vi "Create.vi"(8 "error in (no error)":errorcluster) -> (0 "error out":errorcluster, 3 "GH2 out":refnum<class "GH2.lvclass">)   [LabVIEW 2026, in "GH2.lvclass"]
uses:
  GH2.lvclass
  GH2.lvclass/GH2.ctl
  System.Management
  <vilib>/Instr/_visa.llb/VISA Configure Serial Port (Serial Instr).vi
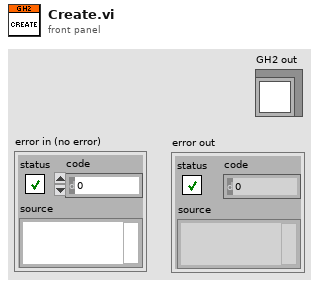
[diagram p1: front panel]
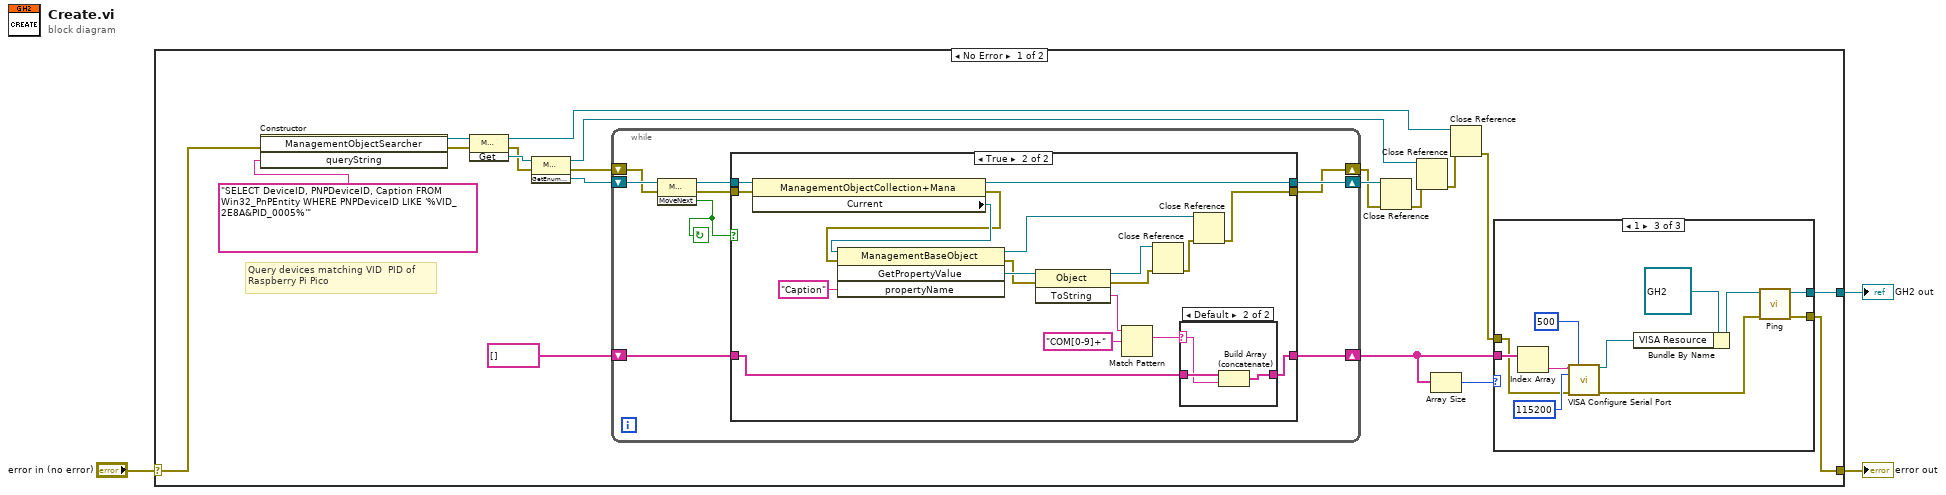
[diagram p0: block diagram]
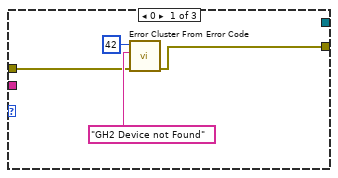
[diagram p2: hidden frame]
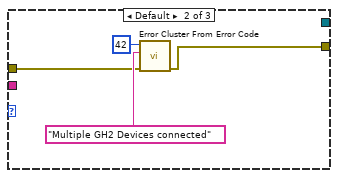
[diagram p3: hidden frame]
diagram:
  n1 = case shown="No Error" "error in (no error)" {
    selector: "error in (no error)" -> [w10 w77]
    tunnel: [w8 w77] -> w2
    tunnel: [w7 _] -> w1
    frame No Error {
      # "Query devices matching VID  PID of\nRaspberry Pi Pico"
      n2 = constructor class="ManagementObjectSearcher"(error in=w10, "queryString"="SELECT DeviceID, PNPDeviceID, Caption FROM Win32_PnPEntity WHERE PNPDeviceID LIKE '%VID_2E8A&PID_0005%'") -> (reference out=w22:refnum<k24>, error out=w17:errorcluster)  [unwired: 2 in, 2 out]
      n3 = invoke class="ManagementObjectSearcher" method="Get"(reference=w22, error in=w17) -> (reference out=w18:refnum<k24>, error out=w16:errorcluster, "Get"=w21:refnum<k24>)  [unwired: 1 in]
      n4 = invoke class="ManagementObjectCollection" method="GetEnumerator"(reference=w21, error in=w16) -> (reference out=w15:refnum<k24>, error out=w14:errorcluster, "GetEnumerator"=w20:refnum<k24>)  [unwired: 1 in]
      n5 = while {
        shift-right: [w48] -> w19
        shift-left: w20 -> [w51]
        shift-right: [w45] -> w13
        shift-left: w14 -> [w47]
        shift-right: [w43] -> w6
        shift-left: string[] [] -> [w44]
        stop <- w50 continue-if-true
        n6 = invoke class="ManagementObjectCollection+Mana" method="MoveNext"(reference=w51, error in=w47) -> (reference out=w49:refnum<k24>, error out=w46:errorcluster, "MoveNext"=w50:bool)  [unwired: 1 in]
        n7 = case shown="True" w50 {
          tunnel: w49 -> [w54 w72]
          tunnel: [w54 w68] -> w48
          tunnel: w46 -> [w53 w66]
          tunnel: [w53 w60] -> w45
          tunnel: w44 -> [w52 w59]
          tunnel: [w52 w56] -> w43
          frame False {
          }
          frame True {
            n8 = property class="ManagementObjectCollection+Mana"(reference=w72, error in=w66) -> (reference out=w68:refnum<k24>, error out=w65:errorcluster, "Current"=w71:refnum<k24>)
            n9 = invoke class="ManagementBaseObject" method="GetPropertyValue"(reference=w71, error in=w65, "propertyName"="Caption") -> (reference out=w67:refnum<k24>, error out=w64:errorcluster, "GetPropertyValue"=w69:refnum<k24>)  [unwired: 1 in, 1 out]
            n10 = invoke class="Object" method="ToString"(reference=w69, error in=w64) -> (reference out=w63:refnum<k24>, error out=w62:errorcluster, "ToString"=w55:string)  [unwired: 1 in]
            n11 = Match Pattern(string=w55, regular expression="COM[0-9]+") -> (match substring=w57:string)  [unwired: 1 in, 3 out]
            n12 = Close Reference(reference=w63, error in (no error)=w62) -> (error out=w61:errorcluster)
            n13 = case shown="Default" w57 {
              selector: w57 -> [_ w74]
              tunnel: w59 -> [w73 w76]
              tunnel: [w73 w75] -> w56
              frame "" {
              }
              frame Default {
                n14 = Build Array (concatenate)(w76, w74) -> (w75:string[])
              }
            }
            n15 = Close Reference(reference=w67, error in (no error)=w61) -> (error out=w60:errorcluster)
          }
        }
      }
      n16 = Close Reference(reference=w19, error in (no error)=w13) -> (error out=w12:errorcluster)
      n17 = Close Reference(reference=w15, error in (no error)=w12) -> (error out=w11:errorcluster)
      n18 = Array Size(array=w6) -> (size(s)=w5:i32)
      n19 = Close Reference(reference=w18, error in (no error)=w11) -> (error out=w4:errorcluster)
      n20 = case shown="1" w5 {
        tunnel: w6 -> [_ _ w42]
        tunnel: [w24 w28 w34] -> w8
        tunnel: [_ _ w33] -> w7
        tunnel: w4 -> [w25 w29 w32]
        frame 0 {
          n21 = call <vilib>:"Error Cluster From Error Code.vi"("error in (no error)"=w25, "error message (\"\")"="GH2 Device not Found" ("error message (\"\")"), "error code (0)"=42) -> ("error out"=w24:errorcluster)  [unwired: 6 in]
        }
        frame Default {
          n22 = call <vilib>:"Error Cluster From Error Code.vi"("error in (no error)"=w29, "error message (\"\")"="Multiple GH2 Devices connected" ("error message (\"\")"), "error code (0)"=42) -> ("error out"=w28:errorcluster)  [unwired: 6 in]
        }
        frame 1 {
          n23 = Index Array(array=w42) -> (element=w41:string)  [unwired: 1 in]
          n24 = call-poly "VISA Configure Serial Port"("VISA resource name"=w41, "timeout (10sec)"=u32 500, "baud rate (9600)"=u32 115200, "error in (no error)"=w32) -> ("VISA resource name out"=w37:refnum<visa-resource-name>, "error out"=w35:errorcluster)  [unwired: 10 in]
          n25 = Bundle By Name(cluster=refnum<class "GH2.lvclass"> refnum ("GH2 in"), "VISA Resource"=w37) -> (w36:refnum<class "GH2.lvclass">)
          n26 = call "Ping.vi"("error in (no error)"=w35, "GH2 in"=w36) -> ("error out"=w34:errorcluster, "GH2 out"=w33:refnum<class "GH2.lvclass">)  [unwired: 8 in]
        }
      }
    }
    frame Error {
    }
  }
  "error out" <- w2
  "GH2 out" <- w1
